vi "Get New Record.vi"(8 "error in (no error)":errorcluster, 11 "Handler.UserEvent in":refnum<class "Handler.UserEvent.lvclass">) -> (0 "error out":errorcluster, 2 "New Record Event":refnum<user-event>, 3 "Handler.UserEvent out":refnum<class "Handler.UserEvent.lvclass">)   [LabVIEW 2017, in "Error Log.lvlib" / "Handler.UserEvent.lvclass"]
uses:
  Handler.UserEvent.lvclass
  Record/Record.lvclass
  Handler.UserEvent.lvclass/Handler.UserEvent.ctl
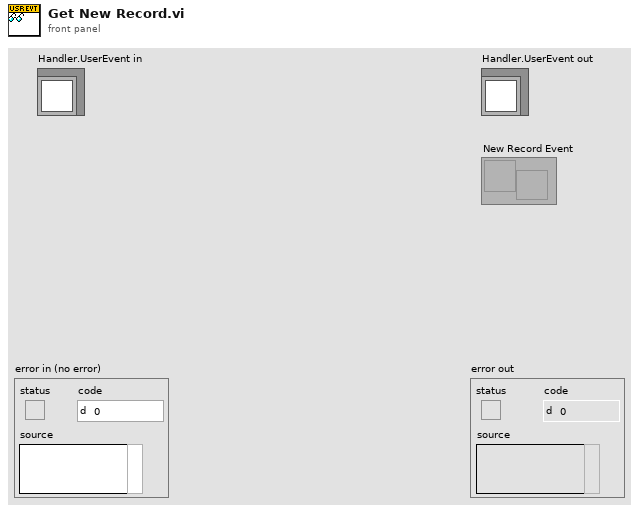
[diagram p1: front panel]
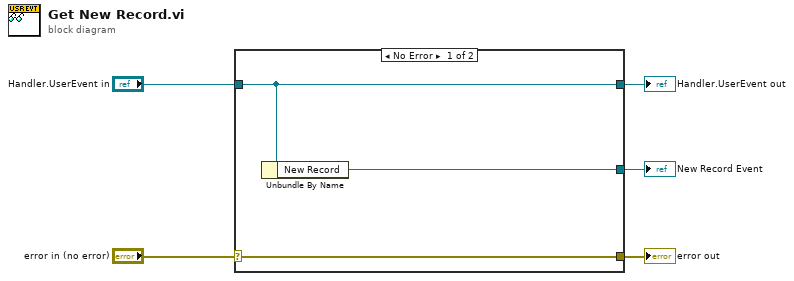
[diagram p0: block diagram]
diagram:
  n1 = case shown="No Error" "error in (no error)" {
    selector: "error in (no error)" -> [w8 w9]
    tunnel: [w8 w9] -> w4
    tunnel: [w7 w10] -> w2
    tunnel: "Handler.UserEvent in" -> [w7 w10]
    tunnel: [w6 _] -> w1
    frame No Error {
      n2 = Unbundle By Name(w7) -> ("New Record"=w6:refnum<user-event>)
    }
    frame Error {
    }
  }
  "error out" <- w4
  "Handler.UserEvent out" <- w2
  "New Record Event" <- w1
